vi "_Main.vi"   [LabVIEW 2017, in "Gimbal.lvlib"]
uses:
  Gimbal.lvlib
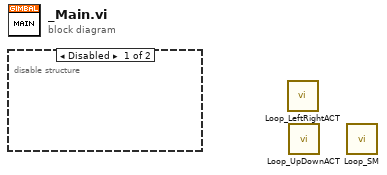
[diagram p0: block diagram]
diagram:
  n1 = disable-structure shown="Disabled" {
    frame Disabled {
    }
    frame Enabled {
    }
  }
  n2 = call "Loop_LeftRightACT.vi"() -> ()  [unwired: 12 in]
  n3 = call "Loop_UpDownACT.vi"() -> ()  [unwired: 12 in]
  n4 = call "Loop_SM.vi"() -> ()  [unwired: 12 in]
